vi "test_CCDOpenAndClose.vi"(7 "Test should pass":bool=TRUE, 8 "error in":errorcluster, 9 "tear down connection":bool=TRUE, 10 "set-up a connection":bool=TRUE, 11 "device selection":enum16{"monochromator", "CCD", "SCD"}(ring)=enum."CCD") -> (0 "error out":errorcluster)   [LabVIEW 2023]
uses:
  Source/Classes/Mono/Monochromator.lvclass
  Source/Classes/CCD/CCD.lvclass
  Source/Classes/SCD/SCD.lvclass
  <vilib>/addons/_JKI Toolkits/Caraya/classes/Assert/Assert Not Error.vi
  Source/Classes/GenericDevice/GenericDevice.lvclass
  <vilib>/addons/_JKI Toolkits/Caraya/classes/Test/Test.lvclass
  <vilib>/addons/_JKI Toolkits/Caraya/classes/Assert/Assert.lvclass
  <vilib>/addons/_JKI Toolkits/Caraya/classes/Assert/Assert Equal Value and Type_Variant.vi
panel:
  # "Connector Pane"
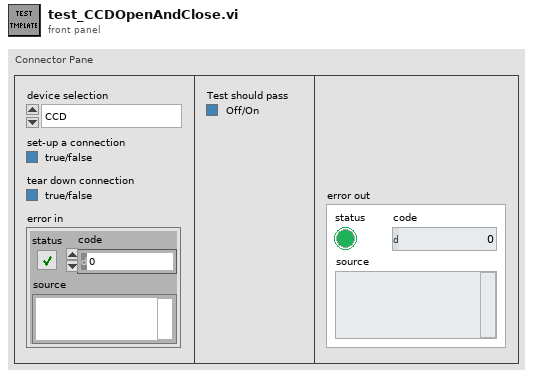
[diagram p1: front panel]
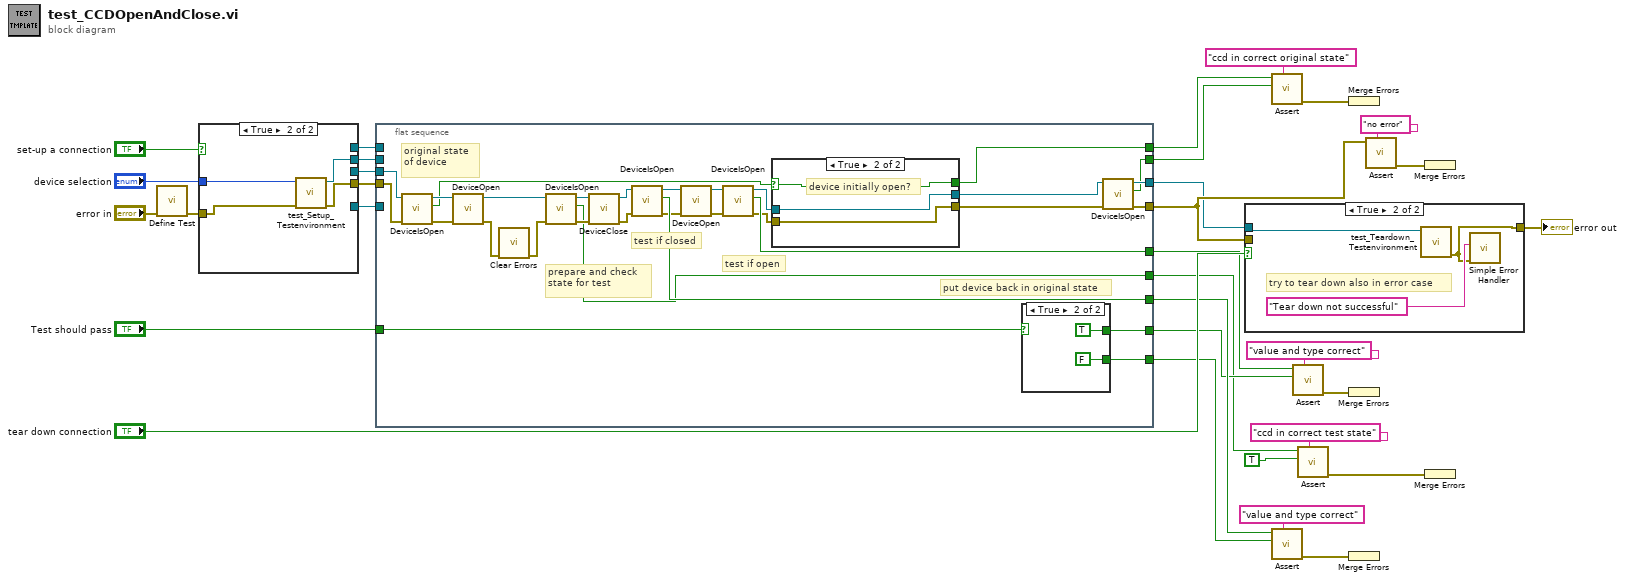
[diagram p0: block diagram]
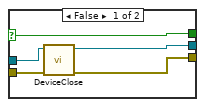
[diagram p2: hidden frame]
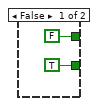
[diagram p3: hidden frame]
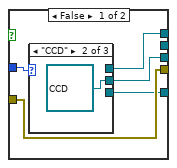
[diagram p5: hidden frame]
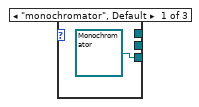
[diagram p6: hidden frame]
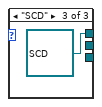
[diagram p7: hidden frame]
diagram:
  n1 = call <vilib>:"Define Test.vi"("error in (no error)"="error in") -> ("error out"=w24:errorcluster)  [unwired: 9 in, 1 out]
  n2 = case shown="True" "set-up a connection" {
    tunnel: w24 -> [w37 w44]
    tunnel: [w37 w43] -> w26
    tunnel: "device selection" -> [w36 w42]
    tunnel: [_ w41] -> w23
    tunnel: [w35 _] -> w22
    tunnel: [w34 _] -> w21
    tunnel: [w33 _] -> w20
    frame False {
      n3 = case shown="\"CCD\"" w36 {
        tunnel: [refnum<class "Monochromator.lvclass"> refnum ("Monochromator.lvclass") _ _] -> w35
        tunnel: [_ refnum<class "CCD.lvclass"> refnum ("CCD in") _] -> w34
        tunnel: [_ _ refnum<class "SCD.lvclass"> refnum ("SCD.lvclass")] -> w33
        frame "monochromator", Default {
        }
        frame "CCD" {
        }
        frame "SCD" {
        }
      }
    }
    frame True {
      n4 = call "test_Setup_Testenvironment.vi"("error in"=w44, "device selection"=w42) -> ("error out"=w43:errorcluster, "GenericDevice.lvclass"=w41:refnum<class "GenericDevice.lvclass">)  [unwired: 7 in, 1 out]
    }
  }
  n5 = flat-sequence {
    tunnel: w26 -> [w73]
    tunnel: w23 -> [_]
    tunnel: w22 -> [_]
    tunnel: w21 -> [w72]
    tunnel: w20 -> [_]
    tunnel: [w48] -> w14
    tunnel: "Test should pass" -> [w74]
    tunnel: [w52] -> w13
    tunnel: [w65] -> w12
    tunnel: [w64] -> w11
    tunnel: [w63] -> w10
    tunnel: [w62] -> w9
    tunnel: [w61] -> w6
    tunnel: [w54] -> w2
    tunnel: [w51] -> w1
    frame #0 {
      # "put device back in original state"
      # "test if open"
      # "test if closed"
      # "original state of device"
      # "prepare and check state for test"
      n6 = call-dynamic "DeviceIsOpen.vi"("error in (no error)"=w73, "CCD in"=w72) -> ("error out"=w47:errorcluster, "device is open?"=w60:bool, "CCD out"=w71:refnum<class "CCD.lvclass">)  [unwired: 6 in, 1 out]
      n7 = call-dynamic "DeviceOpen.vi"("error in (no error)"=w47, "CCD in"=w71) -> ("error out"=w46:errorcluster, "CCD out"=w70:refnum<class "CCD.lvclass">)  [unwired: 6 in, 2 out]
      n8 = call <vilib>:"Clear Errors.vi"("error in (no error)"=w46) -> ("error out"=w45:errorcluster)  [unwired: 5 in, 1 out]
      n9 = call-dynamic "DeviceIsOpen.vi"("error in (no error)"=w45, "CCD in"=w70) -> ("error out"=w66:errorcluster, "device is open?"=w61:bool, "CCD out"=w69:refnum<class "CCD.lvclass">)  [unwired: 6 in, 1 out]
      n10 = call-dynamic "DeviceClose.vi"("error in (no error)"=w66, "CCD in"=w69) -> ("error out"=w67:errorcluster, "CCD out"=w68:refnum<class "CCD.lvclass">)  [unwired: 5 in, 3 out]
      n11 = call-dynamic "DeviceIsOpen.vi"("error in (no error)"=w67, "CCD in"=w68) -> ("error out"=w56:errorcluster, "device is open?"=w65:bool, "CCD out"=w58:refnum<class "CCD.lvclass">)  [unwired: 6 in, 1 out]
      n12 = call-dynamic "DeviceOpen.vi"("error in (no error)"=w56, "CCD in"=w58) -> ("error out"=w55:errorcluster, "CCD out"=w57:refnum<class "CCD.lvclass">)  [unwired: 6 in, 2 out]
      n13 = call-dynamic "DeviceIsOpen.vi"("error in (no error)"=w55, "CCD in"=w57) -> ("error out"=w50:errorcluster, "device is open?"=w63:bool, "CCD out"=w59:refnum<class "CCD.lvclass">)  [unwired: 6 in, 1 out]
      n14 = case shown="True" w60 {
        selector: w60 -> [w77 w80]
        tunnel: w59 -> [w79 w82]
        tunnel: [w78 w82] -> w53
        tunnel: [w77 w80] -> w54
        tunnel: w50 -> [w76 w81]
        tunnel: [w75 w81] -> w49
        frame False {
          n15 = call-dynamic "DeviceClose.vi"("error in (no error)"=w76, "CCD in"=w79) -> ("error out"=w75:errorcluster, "CCD out"=w78:refnum<class "CCD.lvclass">)  [unwired: 5 in, 3 out]
        }
        frame True {
          # "device initially open?"
        }
      }
      n16 = case shown="True" w74 {
        tunnel: [TRUE ("device is open?") FALSE ("device is open?")] -> w64
        tunnel: [FALSE ("device is open?") TRUE ("device is open?")] -> w62
        frame False {
        }
        frame True {
        }
      }
      n17 = call-dynamic "DeviceIsOpen.vi"("error in (no error)"=w49, "CCD in"=w53) -> ("error out"=w48:errorcluster, "device is open?"=w51:bool, "CCD out"=w52:refnum<class "CCD.lvclass">)  [unwired: 6 in, 1 out]
    }
  }
  n18 = case shown="True" "tear down connection" {
    tunnel: w13 -> [_ w89]
    tunnel: [w87 w88] -> w16
    tunnel: w14 -> [w87 _]
    frame False {
    }
    frame True {
      # "try to tear down also in error case"
      n19 = call "test_Teardown_Testenvironment.vi"("GenericDevice.lvclass"=w89) -> ("error out"=w88:errorcluster)  [unwired: 9 in, 1 out]
      n20 = call <vilib>:"Simple Error Handler.vi"("error source (\" \")"="Tear down not successful" ("error source (\" \")"), "error in (no error)"=w88) -> ()  [unwired: 3 in, 5 out]
    }
  }
  "error out" <- w16
  n21 = call-poly <vilib>:"Assert.vi"("Label"="ccd in correct original state" ("Label (VI Title)"), "Y"=w1, "X"=w2) -> ("error out"=w4:errorcluster)  [unwired: 7 in, 1 out]
  n22 = call-poly <vilib>:"Assert.vi"("Label"="value and type correct" ("Label (VI Title)"), "Y"=w11, "X"=w12) -> ("error out"=w30:errorcluster)  [unwired: 7 in, 1 out]
  n23 = call-poly <vilib>:"Assert.vi"("Label"="value and type correct" ("Label (VI Title)"), "Y"=w9, "X"=w10) -> ("error out"=w28:errorcluster)  [unwired: 7 in, 1 out]
  n24 = call-poly <vilib>:"Assert.vi"("Label"="ccd in correct test state" ("Label (VI Title)"), "Y"=TRUE ("device is open?"), "X"=w6) -> ("error out"=w8:errorcluster)  [unwired: 7 in, 1 out]
  n25 = Merge Errors(w4) -> ()  [unwired: 1 out]
  n26 = Merge Errors(w28) -> ()  [unwired: 1 out]
  n27 = Merge Errors(w30) -> ()  [unwired: 1 out]
  n28 = call-poly <vilib>:"Assert.vi"("Label"="no error" ("Label (VI Title)"), "Not Error?"=w14) -> ("error out"=w17:errorcluster)  [unwired: 8 in, 1 out]
  n29 = Merge Errors(w17) -> ()  [unwired: 1 out]
  n30 = Merge Errors(w8) -> ()  [unwired: 1 out]
